vi "0926_2.vi"() -> ()   [LabVIEW 2020]
panel:
  out "병아리반 토익 평균":dbl
  in  "병아리반":T1(array[cluster])
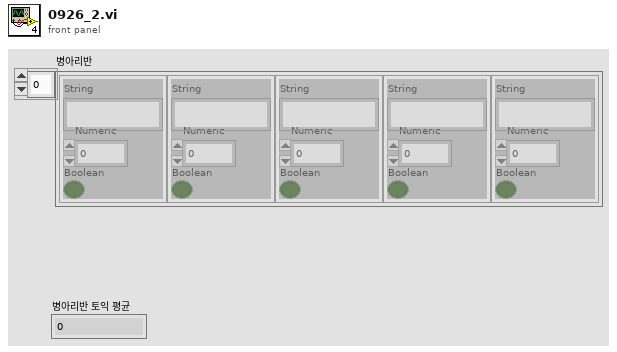
[diagram p1: front panel]
types:
  T1 = cluster{"String":string, "Numeric":dbl, "Boolean":bool}[]
  T2 = cluster{"병아리반[0]":cluster{"String":string, "Numeric":dbl, "Boolean":bool}, "병아리반[1]":cluster{"String":string, "Numeric":dbl, "Boolean":bool}, "병아리반[2]":cluster{"String":string, "Numeric":dbl, "Boolean":bool}, "병아리반[3]":cluster{"String":string, "Numeric":dbl, "Boolean":bool}, "병아리반[4]":cluster{"String":string, "Numeric":dbl, "Boolean":bool}, "병아리반[5]":cluster{"String":string, "Numeric":dbl, "Boolean":bool}, "병아리반[6]":cluster{"String":string, "Numeric":dbl, "Boolean":bool}, "병아리반[7]":cluster{"String":string, "Numeric":dbl, "Boolean":bool}, "병아리반[8]":cluster{"String":string, "Numeric":dbl, "Boolean":bool}}
  T3 = cluster{"String":string, "Numeric":dbl, "Boolean":bool}
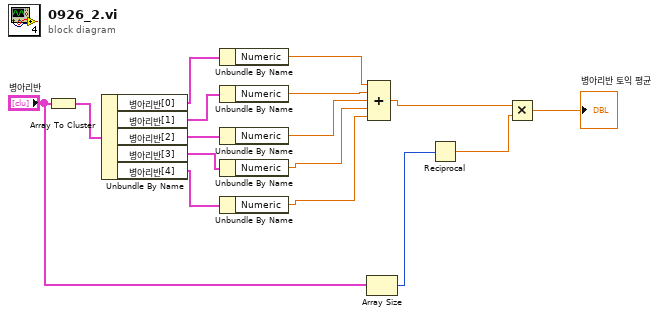
[diagram p0: block diagram]
diagram:
  n1 = Array To Cluster(array="병아리반") -> (cluster=w5:T2)
  n2 = Unbundle By Name(w5) -> ("병아리반[0]"=w15:T3, "병아리반[1]"=w14:T3, "병아리반[2]"=w13:T3, "병아리반[3]"=w12:T3, "병아리반[4]"=w11:T3)
  n3 = Unbundle By Name(w15) -> ("Numeric"=w10:dbl)
  n4 = Unbundle By Name(w14) -> ("Numeric"=w9:dbl)
  n5 = Unbundle By Name(w13) -> ("Numeric"=w8:dbl)
  n6 = Unbundle By Name(w12) -> ("Numeric"=w7:dbl)
  n7 = Unbundle By Name(w11) -> ("Numeric"=w6:dbl)
  n8 = Array Size(array="병아리반") -> (size(s)=w3:i32)
  n9 = Compound Arithmetic op=ADD(w10, w9, w8, w7, w6) -> (w2:dbl)
  n10 = Reciprocal(x=w3) -> (1/x=w16:dbl)
  n11 = Multiply(x=w2, y=w16) -> (x*y=→"병아리반 토익 평균":dbl)
